vi "Line Profile.vi"() -> ()   [LabVIEW 2014]
doc: "This example shows how to use the display tools to draw a line on the window that displays an image and get the pixel values of the image along that line (line profile). You typically use line profiles in inspection and gauging tasks to find the edges of an object or part being inspected."
uses:
  <vilib>/vision/NI_Vision_Development_Module.lvlib
panel:
  in  "Stop":bool
  out "Line Information":T1 {"Standard Deviation" format="%#.2f"; "Mean" format="%#.2f"}
  out "Image":T2(plugin-control)
  out "Line Profile":cluster{"x0":sgl, "dx":sgl, "Pixels Line":sgl[]}(graph)
  # "Overview: Demonstrates how to use the IMAQ LineProfile function to return a line profile of the pixel values along a Region of Interest (ROI).\nRequirements: Vision Development Software.\nInstructions:\n1. Run the VI.\n2. Draw a ROI in the image by left clicking, hold left mouse button down, drag the mouse across the image, and release the mouse button."
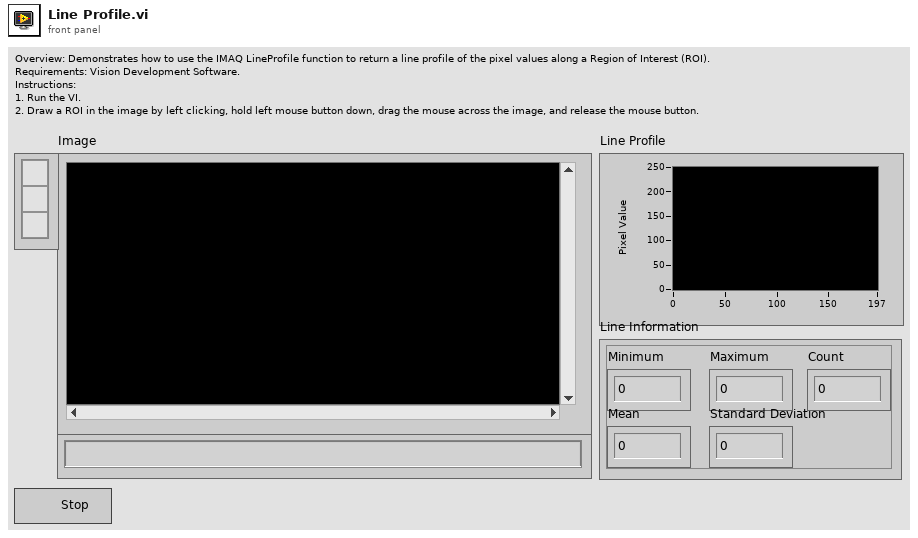
[diagram p1: front panel]
types:
  T1 = cluster{"Minimum":sgl, "Maximum":sgl, "Mean":sgl, "Standard Deviation":sgl, "Count":i32}
  T2 = typedef "IMAQ Image.ctl" = refnum<image>
  T3 = cluster{"Min":sgl, "Max":sgl, "Mean":sgl, "Std Dev":sgl, "Count":i32}
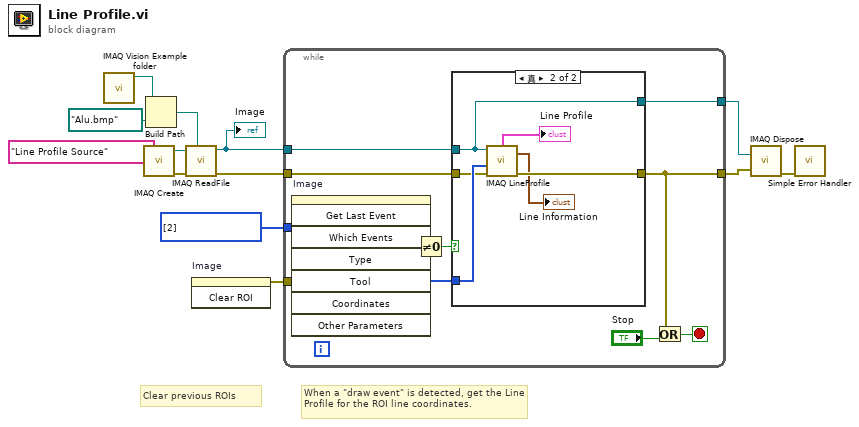
[diagram p0: block diagram]
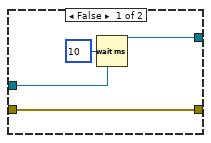
[diagram p2: hidden frame]
diagram:
  w3 = i32[] [2] items=["No  event", "Click event", "Draw event", "Move event", "Size event", "Scroll event", "Activate event", "Close event", "Double click event"] ("Events list (all)")
  # "Clear previous ROIs"
  # "When a \"draw event\" is detected, get the Line Profile for the ROI line coordinates."
  n1 = call "IMAQ Vision Example folder.vi"() -> ("Example Image Path"=w12:path)  [unwired: 11 in]
  n2 = call "IMAQ Create"("Image Name"="Line Profile Source") -> ("New Image"=w11:T2, "error out"=w10:errorcluster)  [unwired: 4 in]
  n3 = Build Path(base path=w12, name or relative path=path "Alu.bmp") -> (appended path=w8:path)
  n4 = call "IMAQ ReadFile"("File Path"=w8, "error in (no error)"=w10, "Image"=w11) -> ("error out"=w7:errorcluster, "Image Out"=w2:T2)  [unwired: 4 in, 3 out]
  "Image" <- w2
  n5 = invoke on="Image" class="ImageControl" method="Clear ROI"() -> (error out=w1:errorcluster)  [unwired: 3 in, 2 out]
  n6 = while {
    tunnel: w2 -> [w21]
    tunnel: w7 -> [w20]
    tunnel: [w16] -> w5
    tunnel: [w22] -> w6
    tunnel: w3 -> [w19]
    tunnel: w1 -> [_]
    stop <- w23 stop-if-true
    n7 = invoke on="Image" class="ImageControl" method="Get Last Event"("Which Events"=w19) -> ("Type"=w18:i32, "Coordinates"=w17:i32[])  [unwired: 7 in, 6 out]
    n8 = Not Equal To 0?(x=w18) -> (x != 0?=w14:bool)
    n9 = case shown="真" w14 {
      tunnel: w21 -> [w25 w29]
      tunnel: [w24 w31] -> w16
      tunnel: [w25 w29] -> w22
      tunnel: w17 -> [_ w32]
      tunnel: w20 -> [w24 w30]
      frame False {
        n10 = Wait (ms)(milliseconds to wait=u32 10) -> ()  [unwired: 1 out]
      }
      frame True {
        n11 = call "IMAQ LineProfile"("error in (no error)"=w30, "Line Coordinates"=w32, "Image"=w29) -> ("error out"=w31:errorcluster, "Line Graph"=→"Line Profile":cluster{"x0":sgl, "dx":sgl, "Pixels Line":sgl[]}, "Line Information"=→"Line Information":T3)  [unwired: 2 in, 1 out]
      }
    }
    n12 = Or(x=w16, y="Stop") -> (x .or. y?=w23:bool)
  }
  n13 = call "IMAQ Dispose"("Image"=w6, "error in (no error)"=w5) -> ("error out"=w4:errorcluster)  [unwired: 4 in]
  n14 = call <vilib>:"Simple Error Handler.vi"("error in (no error)"=w4) -> ()  [unwired: 4 in, 5 out]
